vi "background writer.vi"(0 "dictionary":T2, 1 "logging path":path, 2 "backup directory":path, 3 "output type order":T4[](array[typedef]), 4 "cache allocation":T3, 5 "scans per write":i32=20, 6 "command queue":refnum<queue>, 7 "group name":string, 8 "error q":refnum<queue>, 9 "has enable channel":bool, 10 "from background":refnum<queue>, 11 "enable channel (bool)":i32, 12 "sample queue":T1) -> (19 "error out":errorcluster)   [LabVIEW 2013, in "TDMS datalogger runtime.lvclass"]
uses:
  TDMS datalogger runtime.lvclass
  <vilib>/NI/Tag Bus/tag/Data Type.ctl
  <vilib>/NI/Tag Bus/table/data table.ctl
  control enum.ctl
  data cache.ctl
  <vilib>/NI/Tag Bus/dictionary/full data dictionary.ctl
  sample queue.ctl
  writer state enum.ctl
  move to cache.vi
  write cache to tdms.vi
  <vilib>/NI/Tag Bus/tag/tag descriptor.lvclass
  <vilib>/NI/Tag Bus/table/data table.lvlib
  <vilib>/NI/Tag Bus/dictionary/data dictionary.lvclass
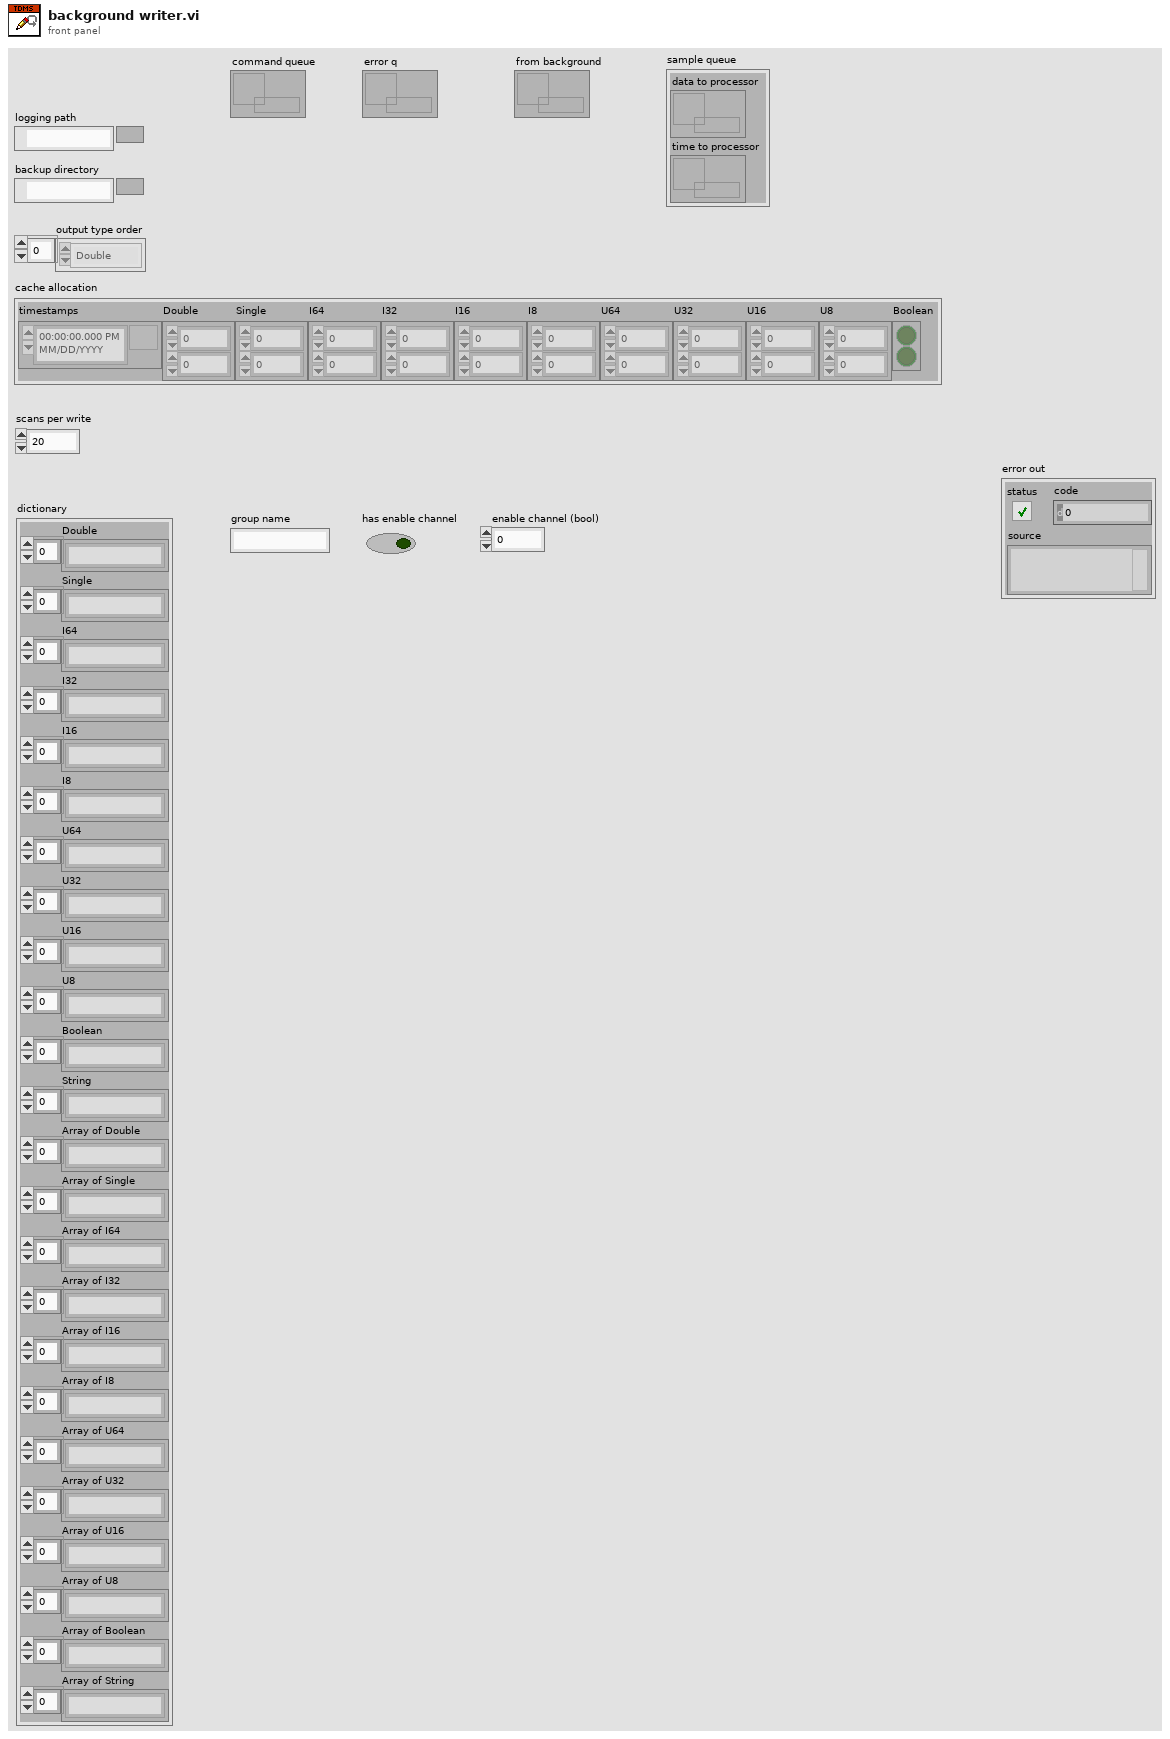
[diagram p1: front panel]
types:
  T1 = typedef "TDMS datalogger runtime.lvclass/sample queue.ctl" = cluster{"data to processor":refnum<queue>, "time to processor":refnum<queue>}
  T2 = typedef "tag bus.lvlib/data dictionary.lvclass/full data dictionary.ctl" = cluster{"Double":string[], "Single":string[], "I64":string[], "I32":string[], "I16":string[], "I8":string[], "U64":string[], "U32":string[], "U16":string[], "U8":string[], "Boolean":string[], "String":string[], "Array of Double":string[], "Array of Single":string[], "Array of I64":string[], "Array of I32":string[], "Array of I16":string[], "Array of I8":string[], "Array of U64":string[], "Array of U32":string[], "Array of U16":string[], "Array of U8":string[], "Array of Boolean":string[], "Array of String":string[]}
  T3 = typedef "TDMS datalogger runtime.lvclass/data cache.ctl" = cluster{"timestamps":timestamp[], "Double":dbl[][], "Single":sgl[][], "I64":i64[][], "I32":i32[][], "I16":i16[][], "I8":i8[][], "U64":u64[][], "U32":u32[][], "U16":u16[][], "U8":u8[][], "Boolean":bool[][]}
  T4 = typedef "tag bus.lvlib/tag descriptor.lvclass/Data Type.ctl" = enum16{"Double", "Single", "I64", "I32", "I16", "I8", "U64", "U32", "U16", "U8", "Boolean", "String", "Array of Double", "Array of Single", "Array of I64", "Array of I32", "Array of I16", "Array of I8", "Array of U64", "Array of U32", "Array of U16", "Array of U8", "Array of Boolean", "Array of String"}
  T5 = typedef "TDMS datalogger runtime.lvclass/writer state enum.ctl" = enum16{"idle", "initialize file", "running", "close file", "stopping"}
  T6 = typedef "TDMS datalogger runtime.lvclass/control enum.ctl" = enum16{"exit"}
  T7 = typedef "tag bus.lvlib/data table.lvlib/data table.ctl" = cluster{"Double":dbl[], "Single":sgl[], "I64":i64[], "I32":i32[], "I16":i16[], "I8":i8[], "U64":u64[], "U32":u32[], "U16":u16[], "U8":u8[], "Boolean":bool[], "String":string[], "Array of Double":cluster{"DBL Array":dbl[]}[], "Array of Single":cluster{"SGL Array":sgl[]}[], "Array of I64":cluster{"I64 Array":i64[]}[], "Array of I32":cluster{"I32 Array":i32[]}[], "Array of I16":cluster{"I16 Array":i16[]}[], "Array of I8":cluster{"I8 Array":i8[]}[], "Array of U64":cluster{"U64 Array":u64[]}[], "Array of U32":cluster{"U32 Array":u32[]}[], "Array of U16":cluster{"U16 Array":u16[]}[], "Array of U8":cluster{"U8 Array":u8[]}[], "Array of Boolean":cluster{"Boolean Array":bool[]}[], "Array of String":cluster{"String Array":string[]}[]}
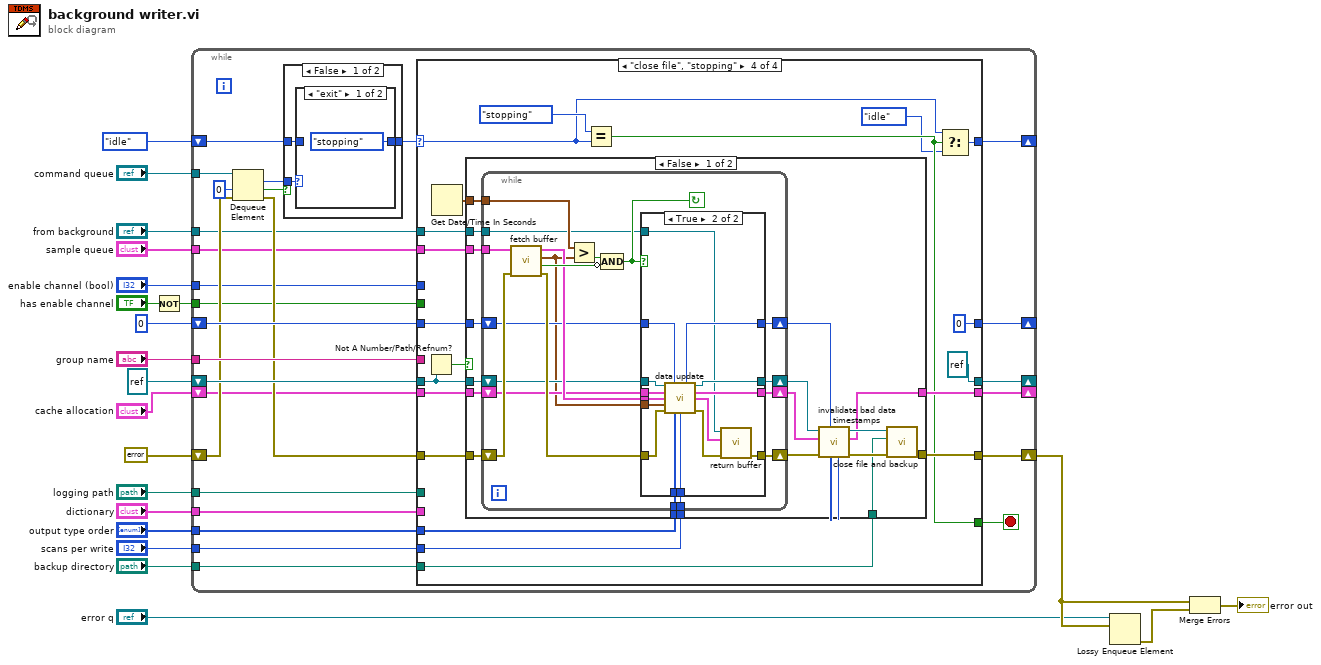
[diagram p0: block diagram]
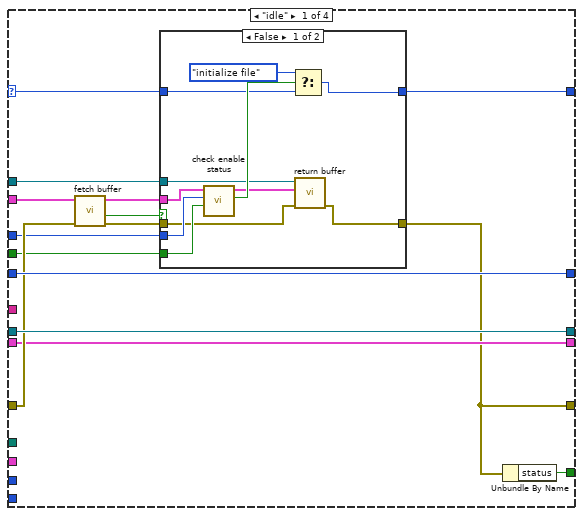
[diagram p4: hidden frame]
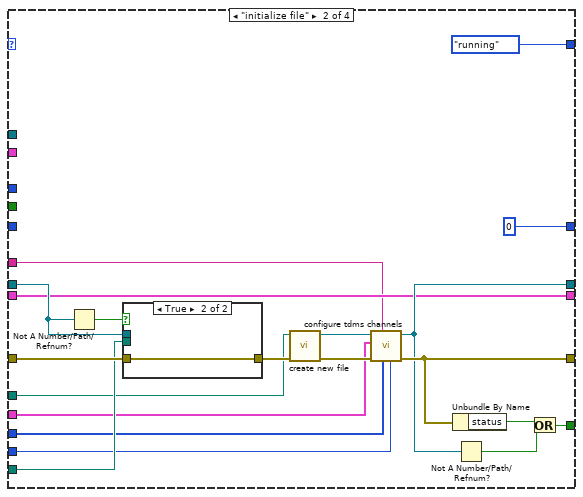
[diagram p6: hidden frame]
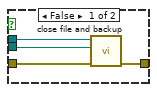
[diagram p7: hidden frame]
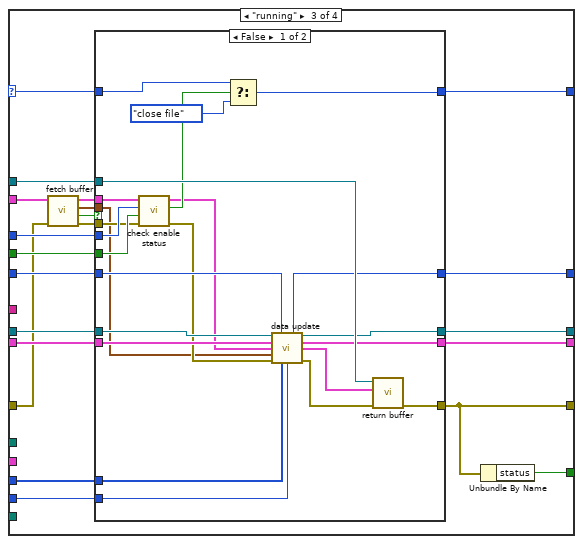
[diagram p8: hidden frame]
diagram:
  n1 = Not(x="has enable channel") -> (.not. x?=w5:bool)
  n2 = while {
    tunnel: "command queue" -> [w32]
    shift-right: [w46] -> _
    shift-left: writer_state_enum."idle" ("logger state") -> [w29]
    shift-right: [w48] -> w9
    shift-left: errorcluster {"status"=FALSE, "code"=0, "source"=""} ("error in") -> [w34]
    shift-right: [w38] -> _
    shift-left: refnum<k34> refnum ("tdms file out") -> [w45]
    tunnel: "backup directory" -> [w44]
    tunnel: "logging path" -> [w43]
    tunnel: "group name" -> [w42]
    tunnel: "dictionary" -> [w41]
    tunnel: "output type order" -> [w40]
    tunnel: "scans per write" -> [w39]
    shift-right: [w37] -> _
    shift-left: 0 ("sample counter") -> [w36]
    tunnel: "sample queue" -> [w27]
    tunnel: "from background" -> [w26]
    tunnel: w5 -> [w24]
    tunnel: "enable channel (bool)" -> [w25]
    shift-right: [w23] -> _
    shift-left: "cache allocation" -> [w22]
    stop <- w47 stop-if-true
    n3 = Dequeue Element(queue=w32, timeout in ms (-1)=0, error in (no error)=w34) -> (element=w30:T6, timed out?=w31:bool, error out=w33:errorcluster)  [unwired: 1 out]
    n4 = case shown="False" w31 {
      tunnel: w30 -> [w51 _]
      tunnel: w29 -> [w49 w54]
      tunnel: [w50 w54] -> w28
      frame False {
        n5 = case shown="\"exit\"" w51 {
          tunnel: [writer_state_enum."stopping" ("logger state") w53] -> w50
          tunnel: w49 -> [_ w53]
          frame "exit" {
          }
          frame Default {
          }
        }
      }
      frame True {
      }
    }
    n6 = case shown="\"close file\", \"stopping\"" w28 {
      selector: w28 -> [w64 _ w127 w160]
      tunnel: w33 -> [w66 w101 w116 w173]
      tunnel: [w57 w89 w111 w168] -> w48
      tunnel: [w56 w90 w110 w161] -> w47
      tunnel: [w65 writer_state_enum."running" ("logger state") w128 w158] -> w46
      tunnel: w45 -> [w69 w98 w123 w157]
      tunnel: w44 -> [_ w100 _ w163]
      tunnel: w43 -> [_ w96 _ _]
      tunnel: w42 -> [_ w83 _ _]
      tunnel: w41 -> [_ w94 _ _]
      tunnel: w40 -> [_ w85 w113 w166]
      tunnel: w39 -> [_ w84 w112 w165]
      tunnel: [w69 w88 w122 refnum<k34> refnum ("tdms file out")] -> w38
      tunnel: [w68 0 ("sample counter") w118 0 ("sample counter")] -> w37
      tunnel: w36 -> [w68 _ w119 w171]
      tunnel: w27 -> [w67 _ w117 w175]
      tunnel: w26 -> [w63 _ w126 w172]
      tunnel: w25 -> [w60 _ w125 _]
      tunnel: w24 -> [w59 _ w124 _]
      tunnel: [w58 w86 w121 w164] -> w23
      tunnel: w22 -> [w58 w86 w120 w170]
      frame "idle" {
        n7 = call "fetch buffer.vi"("error in"=w66, "sample queue"=w67) -> ("error out"=w62:errorcluster, "empty?"=w55:bool, "data table"=w61:T7)  [unwired: 6 in, 1 out]
        n8 = case shown="False" w55 {
          tunnel: [w74 w82] -> w65
          tunnel: w64 -> [w76 w82]
          tunnel: w63 -> [w72 _]
          tunnel: w62 -> [w70 w81]
          tunnel: [w73 w81] -> w57
          tunnel: w61 -> [w80 _]
          tunnel: w60 -> [w78 _]
          tunnel: w59 -> [w79 _]
          frame False {
            n9 = call "check enable status.vi"("always enabled?"=w79, "enable channel index"=w78, "data table in"=w80) -> ("enabled?"=w77:bool, "Data table out"=w71:T7)  [unwired: 7 in]
            n10 = Select(t=writer_state_enum."initialize file", s=w77, f=w76) -> (s? t:f=w74:T5)
            n11 = call "return buffer.vi"("error in (no error)"=w70, "data table in"=w71, "Queue in"=w72) -> ("error out"=w73:errorcluster)  [unwired: 8 in]
          }
          frame True {
          }
        }
        n12 = Unbundle By Name(w57) -> ("status"=w56:bool)
      }
      frame "initialize file" {
        n13 = Not A Number/Path/Refnum?(number/path/refnum=w98) -> (NaN/Path/Refnum?=w99:bool)
        n14 = case shown="True" w99 {
          tunnel: [w105 w107] -> w97
          tunnel: w101 -> [w106 w107]
          tunnel: w98 -> [w104 _]
          tunnel: w100 -> [w103 _]
          frame False {
            n15 = call "close file and backup.vi"("error in"=w106, "backup directory"=w103, "tdms file in"=w104) -> ("error out"=w105:errorcluster)  [unwired: 8 in]
          }
          frame True {
          }
        }
        n16 = call "create new file.vi"("error in"=w97, "logging path"=w96) -> ("error out"=w95:errorcluster, "tdms file out"=w93:refnum<k34>)  [unwired: 8 in]
        n17 = call "configure tdms channels.vi"("samples per channel (1)"=w84, "type order"=w85, "group name"=w83, "error in"=w95, "dictionary"=w94, "tdms file in"=w93) -> ("error out"=w89:errorcluster, "tdms file out"=w88:refnum<k34>)  [unwired: 4 in]
        n18 = Unbundle By Name(w89) -> ("status"=w91:bool)
        n19 = Not A Number/Path/Refnum?(number/path/refnum=w88) -> (NaN/Path/Refnum?=w92:bool)
        n20 = Or(x=w91, y=w92) -> (x .or. y?=w90:bool)
      }
      frame "running" {
        n21 = call "fetch buffer.vi"("error in"=w116, "sample queue"=w117) -> ("error out"=w115:errorcluster, "empty?"=w109:bool, "Time Stamp"=w108:timestamp, "data table"=w114:T7)  [unwired: 6 in]
        n22 = case shown="False" w109 {
          tunnel: [w144 w155] -> w128
          tunnel: w127 -> [w134 w155]
          tunnel: w126 -> [w147 _]
          tunnel: w115 -> [w130 w154]
          tunnel: [w146 w154] -> w111
          tunnel: w114 -> [w150 _]
          tunnel: w125 -> [w148 _]
          tunnel: w124 -> [w149 _]
          tunnel: w123 -> [w143 w152]
          tunnel: [w142 w152] -> w122
          tunnel: [w141 w151] -> w121
          tunnel: w120 -> [w140 w151]
          tunnel: w119 -> [w139 w153]
          tunnel: [w138 w153] -> w118
          tunnel: w113 -> [w132 _]
          tunnel: w112 -> [w131 _]
          tunnel: w108 -> [w129 _]
          frame False {
            n23 = call "check enable status.vi"("always enabled?"=w149, "enable channel index"=w148, "data table in"=w150) -> ("enabled?"=w145:bool, "Data table out"=w137:T7)  [unwired: 7 in]
            n24 = Select(t=w134, s=w145, f=writer_state_enum."close file" ("t")) -> (s? t:f=w144:T5)
            n25 = call "data update.vi"("tdms in"=w143, "sample counter in"=w139, "cache in"=w140, "data table in"=w137, "Time Stamp"=w129, "error in"=w130, "output type order"=w132, "scans per write"=w131) -> ("sample counter out"=w138:i32, "tdms out"=w142:refnum<k34>, "cache out"=w141:T3, "data table out"=w136:T7, "error out"=w135:errorcluster)  [unwired: 3 in]
            n26 = call "return buffer.vi"("error in (no error)"=w135, "data table in"=w136, "Queue in"=w147) -> ("error out"=w146:errorcluster)  [unwired: 8 in]
          }
          frame True {
          }
        }
        n27 = Unbundle By Name(w111) -> ("status"=w110:bool)
      }
      frame "close file", "stopping" {
        n28 = Not A Number/Path/Refnum?(number/path/refnum=w157) -> (NaN/Path/Refnum?=w156:bool)
        n29 = Get Date/Time In Seconds() -> (seconds since 1Jan1904=w174:timestamp)
        n30 = case shown="False" w156 {
          tunnel: w175 -> [w193 _]
          tunnel: w174 -> [w192 _]
          tunnel: w173 -> [w191 w232]
          tunnel: w172 -> [w190 _]
          tunnel: w171 -> [w189 _]
          tunnel: w170 -> [w188 w233]
          tunnel: [w185 w232] -> w168
          tunnel: w166 -> [w180 _]
          tunnel: w165 -> [w179 _]
          tunnel: [w178 w233] -> w164
          tunnel: w163 -> [w177 _]
          tunnel: w157 -> [w176 _]
          frame False {
            n31 = while {
              tunnel: w193 -> [w212]
              tunnel: w192 -> [w210]
              shift-right: [w199] -> w181
              shift-left: w191 -> [w211]
              tunnel: w190 -> [w206]
              shift-right: [w202] -> w184
              shift-left: w176 -> [w203]
              shift-right: [w197] -> w182
              shift-left: w189 -> [w198]
              shift-right: [w200] -> w183
              shift-left: w188 -> [w201]
              tunnel: w180 -> [w196]
              tunnel: w179 -> [w195]
              stop <- w207 continue-if-true
              n32 = call "fetch buffer.vi"("error in"=w211, "sample queue"=w212) -> ("error out"=w205:errorcluster, "empty?"=w209:bool, "Time Stamp"=w194:timestamp, "data table"=w204:T7)  [unwired: 6 in]
              n33 = Greater?(x=w210, y=w194) -> (0:w208:bool)
              n34 = Compound Arithmetic op=AND(w208, invert w209) -> (w207:bool)
              n35 = case shown="True" w207 {
                tunnel: w206 -> [_ w219]
                tunnel: w205 -> [w214 w221]
                tunnel: w204 -> [_ w227]
                tunnel: w203 -> [w216 w231]
                tunnel: [w216 w229] -> w202
                tunnel: w201 -> [w215 w230]
                tunnel: [w215 w228] -> w200
                tunnel: [w214 w220] -> w199
                tunnel: w198 -> [w213 w224]
                tunnel: [w213 w223] -> w197
                tunnel: w196 -> [_ w226]
                tunnel: w195 -> [_ w225]
                tunnel: w194 -> [_ w222]
                frame False {
                }
                frame True {
                  n36 = call "data update.vi"("tdms in"=w231, "sample counter in"=w224, "cache in"=w230, "data table in"=w227, "Time Stamp"=w222, "error in"=w221, "output type order"=w226, "scans per write"=w225) -> ("sample counter out"=w223:i32, "tdms out"=w229:refnum<k34>, "cache out"=w228:T3, "data table out"=w218:T7, "error out"=w217:errorcluster)  [unwired: 3 in]
                  n37 = call "return buffer.vi"("error in (no error)"=w217, "data table in"=w218, "Queue in"=w219) -> ("error out"=w220:errorcluster)  [unwired: 8 in]
                }
              }
            }
            n38 = call "invalidate bad data timestamps.vi"("scans per write"=w179, "output type order"=w180, "sample counter"=w182, "error in"=w181, "cache allocation in"=w183, "tdms file in"=w184) -> ("error out"=w187:errorcluster, "cache allocation out"=w178:T3, "tdms file out"=w186:refnum<k34>)  [unwired: 3 in]
            n39 = call "close file and backup.vi"("error in"=w187, "backup directory"=w177, "tdms file in"=w186) -> ("error out"=w185:errorcluster)  [unwired: 8 in]
          }
          frame True {
          }
        }
        n40 = Equal?(x=writer_state_enum."stopping" ("logger state"), y=w160) -> (x = y?=w161:bool)
        n41 = Select(t=w160, s=w161, f=writer_state_enum."idle") -> (s? t:f=w158:T5)
      }
    }
  }
  n42 = Lossy Enqueue Element(queue="error q", element=w9) -> (error out=w20:errorcluster)  [unwired: 1 in, 3 out]
  n43 = Merge Errors(w9, w20) -> (→"error out":errorcluster)
